vi "test.workspace_create_datasource_and_connection_specifying_default_workspace.vi"   [LabVIEW 2020]
uses:
  730c9c5b-7bb2-47cf-818b-6e2ed47344d4.vi
  Nominal Client/Nominal Client.lvclass
  <vilib>/addons/_JKI Toolkits/Caraya/classes/Test/Test.lvclass
  <vilib>/addons/_JKI Toolkits/Caraya/classes/Assert/Assert.lvclass
  7b397072-28d8-4cad-b009-c353cc64c800.vi
  <vilib>/addons/_JKI Toolkits/Caraya/classes/Assert/Assert Not Error.vi
  <vilib>/addons/_JKI Toolkits/Caraya/classes/Assert/Assert Error.vi
  <vilib>/addons/_JKI Toolkits/Caraya/classes/Assert/Assert True.vi
  nominal types/workspace/workspace.lvclass
  C:/code/labview-client/lv_src/nominal types/workspace/workspace.lvclass
  C:/code/labview-client/lv_src/datasources/payload/payload.lvclass
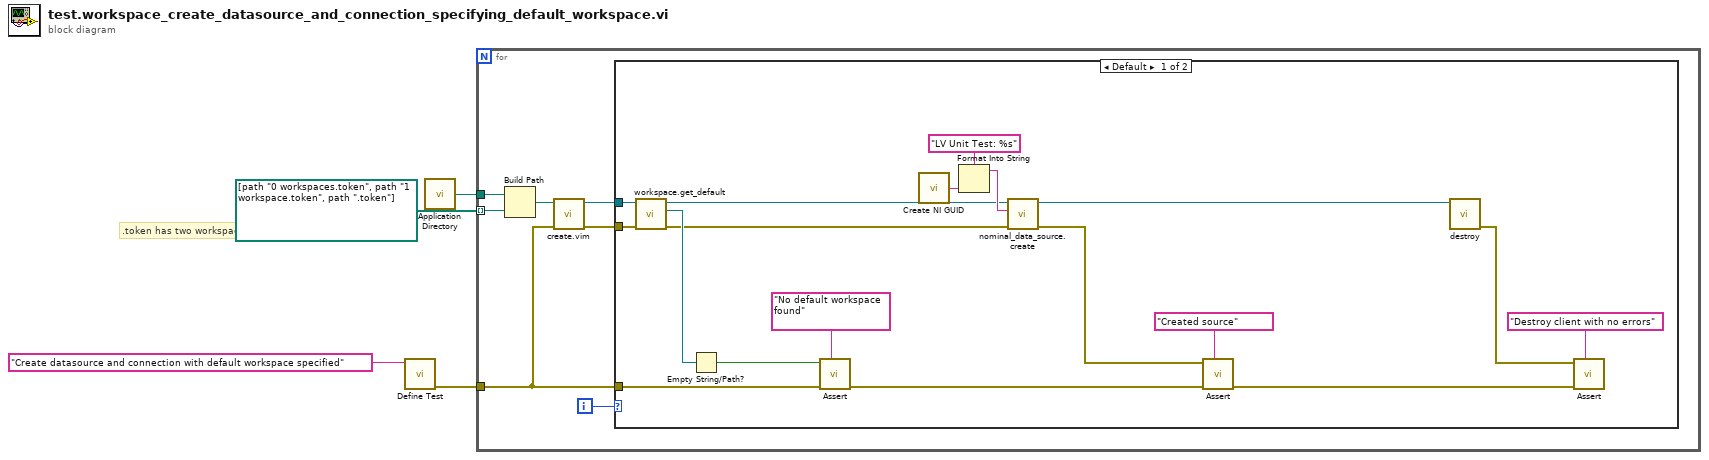
[diagram p0: block diagram]
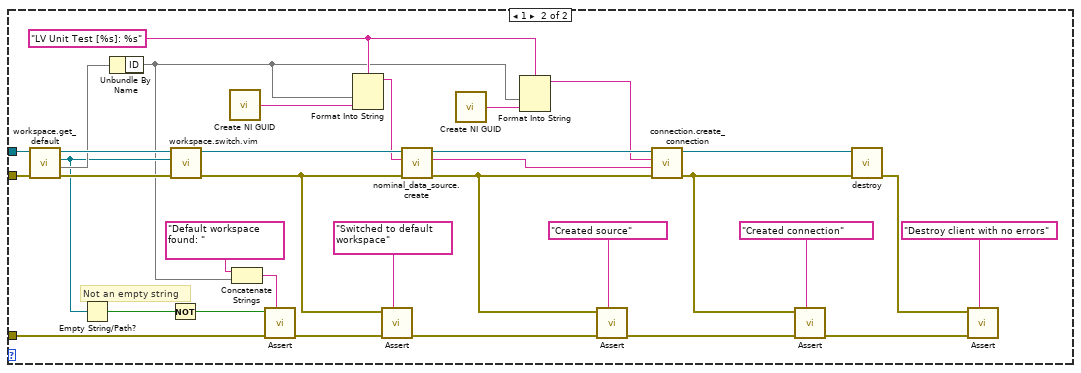
[diagram p2: hidden frame]
diagram:
  # ".token has two workspaces"
  n1 = call <vilib>:"Define Test.vi"("Label (VI Title)"="Create datasource and connection with default workspace specified") -> ("error out"=w3:errorcluster)  [unwired: 9 in, 1 out]
  n2 = call <vilib>:"Application Directory.vi"() -> ("Application Directory"=w2:path)
  n3 = for {
    tunnel: w3 -> [w9]
    tunnel: w2 -> [w8]
    tunnel: path[] [path "0 workspaces.token", path "1 workspace.token", path ".token"] -> [w7] mode=indexing
    i -> [w5]
    n4 = Build Path(base path=w8, name or relative path=w7) -> (appended path=w6:path)
    n5 = call "create.vim"("error in"=w9, "API Token (string or path)"=w6) -> ("error out"=w10:errorcluster, "Nominal Client"=w11:refnum<class "Nominal Client.lvclass">)  [unwired: 7 in, 1 out]
    n6 = case shown="Default" w5 {
      tunnel: w11 -> [w27 w55]
      tunnel: w10 -> [w26 w52]
      tunnel: w9 -> [w23 w42]
      frame Default {
        n7 = call "workspace.get_default.vi"("error in"=w26, "Nominal Client in"=w27) -> ("error out"=w16:errorcluster, "Workspace"=w19:refnum<class "workspace.lvclass">, "Nominal Client out"=w17:refnum<class "Nominal Client.lvclass">)  [unwired: 7 in]
        n8 = Empty String/Path?(string/path=w19) -> (empty?=w18:bool)
        n9 = call-poly <vilib>:"Assert.vi"("Label"="No default workspace found", "error in (no error)"=w23, "True?"=w18) -> ("error out"=w13:errorcluster)  [unwired: 7 in, 1 out]
        n10 = call <vilib>:"Create NI GUID.vi"() -> ("NI GUID"=w14:string)
        n11 = Format Into String(format string="LV Unit Test: %s", w14) -> (resulting string=w25:string)  [unwired: 2 in, 1 out]
        n12 = call "nominal_data_source.create.vi"("error in"=w16, "Name"=w25, "Nominal Client in"=w17) -> ("error out"=w21:errorcluster, "Nominal Client out"=w15:refnum<class "Nominal Client.lvclass">)  [unwired: 5 in, 2 out]
        n13 = call-poly <vilib>:"Assert.vi"("Label"="Created source", "error in (no error)"=w13, "Error?"=w21) -> ("error out"=w12:errorcluster)  [unwired: 7 in, 1 out]
        n14 = call "destroy.vi"("Nominal Client"=w15) -> ("error out"=w29:errorcluster)  [unwired: 10 in]
        n15 = call-poly <vilib>:"Assert.vi"("Label"="Destroy client with no errors", "error in (no error)"=w12, "Not Error?"=w29) -> ()  [unwired: 7 in, 2 out]
      }
      frame 1 {
        w45 = "LV Unit Test [%s]: %s" ("format string")
        # "Not an empty string"
        n16 = call "workspace.get_default.vi"("error in"=w52, "Nominal Client in"=w55) -> ("error out"=w53:errorcluster, 1:w50, "Workspace"=w44:refnum<class "workspace.lvclass">, "Nominal Client out"=w54:refnum<class "Nominal Client.lvclass">)  [unwired: 6 in]
        n17 = Empty String/Path?(string/path=w44) -> (empty?=w43:bool)
        n18 = Unbundle By Name(w50) -> ("ID"=w40)
        n19 = Not(x=w43) -> (.not. x?=w38:bool)
        n20 = call "workspace.switch.vim"("error in"=w53, "Workspace (Object, RID, Path)"=w44, "Nominal Client in"=w54) -> ("error out"=w33:errorcluster, "Nominal Client out"=w51:refnum<class "Nominal Client.lvclass">)  [unwired: 7 in]
        n21 = call <vilib>:"Create NI GUID.vi"() -> ("NI GUID"=w49:string)
        n22 = Concatenate Strings("Default workspace found: " ("Label"), w40) -> (w39:string)
        n23 = call-poly <vilib>:"Assert.vi"("Label"=w39, "error in (no error)"=w42, "True?"=w38) -> ("error out"=w32:errorcluster)  [unwired: 7 in, 1 out]
        n24 = Format Into String(format string=w45, w40, w49) -> (resulting string=w48:string)  [unwired: 2 in, 1 out]
        n25 = call-poly <vilib>:"Assert.vi"("Label"="Switched to default workspace", "error in (no error)"=w32, "Not Error?"=w33) -> ("error out"=w31:errorcluster)  [unwired: 7 in, 1 out]
        n26 = call "nominal_data_source.create.vi"("error in"=w33, "Name"=w48, "Nominal Client in"=w51) -> ("error out"=w36:errorcluster, "rid"=w57:string, "Nominal Client out"=w58:refnum<class "Nominal Client.lvclass">)  [unwired: 5 in, 1 out]
        n27 = call <vilib>:"Create NI GUID.vi"() -> ("NI GUID"=w47:string)
        n28 = Format Into String(format string=w45, w40, w47) -> (resulting string=w46:string)  [unwired: 2 in, 1 out]
        n29 = call-poly <vilib>:"Assert.vi"("Label"="Created source", "error in (no error)"=w31, "Not Error?"=w36) -> ("error out"=w56:errorcluster)  [unwired: 7 in, 1 out]
        n30 = call "connection.create_connection.vi"("error in"=w36, "nominalDataSourceRid"=w57, "name"=w46, "Nominal Client in"=w58) -> ("error out"=w30:errorcluster, "Nominal Client out"=w60:refnum<class "Nominal Client.lvclass">)  [unwired: 4 in, 2 out]
        n31 = call-poly <vilib>:"Assert.vi"("Label"="Created connection", "error in (no error)"=w56, "Not Error?"=w30) -> ("error out"=w59:errorcluster)  [unwired: 7 in, 1 out]
        n32 = call "destroy.vi"("error in"=w30, "Nominal Client"=w60) -> ("error out"=w62:errorcluster)  [unwired: 9 in]
        n33 = call-poly <vilib>:"Assert.vi"("Label"="Destroy client with no errors", "error in (no error)"=w59, "Not Error?"=w62) -> ()  [unwired: 7 in, 2 out]
      }
    }
  }
